vi "MCCDAQ.vi"() -> (0 "error out":errorcluster)   [LabVIEW 2020]
uses:
  Globals/Meas_global.vi
  <vilib>/ULx/Create Channel.llb/ULx Create Channel (AI-Voltage-Basic).vi
  <vilib>/ULx/Timing.llb/ULx Timing (Sample Clock).vi
  <vilib>/ULx/Read.llb/ULx Read (Analog 2D DBL NChan NSamp).vi
  C:/Program Files (x86)/National Instruments/LabVIEW 2020/vi.lib/ULx/ULx_LV.dll
  Sub_vis/Upload Data.ctl
panel:
  out "format string":string
  out "DeviceName":string
  out "FsReq":dbl
  out "FsRead":dbl format="%#_11g"
  out "AuditTrail":string[](array[string])
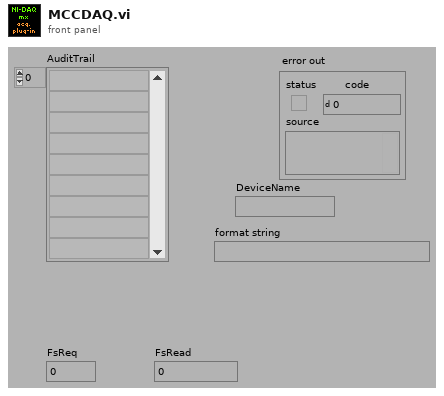
[diagram p1: front panel]
types:
  T1 = typedef "Analysis_info_cluster.ctl" = cluster{"Colour":u32, "Inst type":T2, "Inst name":string, "Symbol":string, "Code name":string, "Extra Info":string, "Inst Array":T3, "Extra Titles":string[], "Extra Values":string[], "U":dbl, "u^2":dbl, "u^3":dbl, "u^4":dbl, "Skew_u":dbl, "Kurt_u":dbl, "Sd Error in Mean":dbl, "% u'/U":dbl, "X":dbl, "Y":dbl, "Z":dbl, "Timescale integral Estimate":dbl, "Sd Error in Variance":dbl, "Calib File":path, "Calib Constants":dbl[], "Output Position":bool, "Stats":enum16{"None", "Basic", "Full"}, "Av Sampling Rate":dbl, "Av No of Samples":dbl, "Total Meas Time (s)":dbl, "ADAM Ch Name":string, "Max value":dbl, "Min value":dbl, "Req Sample Rate Hz":dbl, "Sync Delay Time (s)":dbl, "Ch No":i16, "Device":string, "Use Latest Calib":bool, "Port":string, "Metadata Ch Names":string[], "Metadata Ch Values":string[], "Label":string}
  T2 = typedef "Inst_type.ctl" = enum16{"Raw voltage", "Raw with zero offsetting", "Propeller anemometer", "Pressure Transducer", "Pitot-static tube", "Hot wire", "Cross wire 1", "Cross wire 2", "Generic Linear", "Generic Polynomial", "Generic BackPoly", "Fast FID", "Thermocouple", "Cold wire", "Pulsed Wire", "LDA Vel", "LDA Tran time", "LDA Arr time", "Microphone"}
  T3 = typedef "Instrument_Array.ctl" = enum16{"PWA", "LDA", "Analogue"}
  T4 = typedef "Device ID port info.ctl" = cluster{"Ch No":i16[], "Req Sampling Rate":dbl[], "Port":string, "Index":i32[]}
  T5 = typedef "Upload Data.ctl" = enum16{"Voltage Array", "Time Trace Cluster"}
  T6 = typedef "Rendezvous RefNum" = refnum<k1>
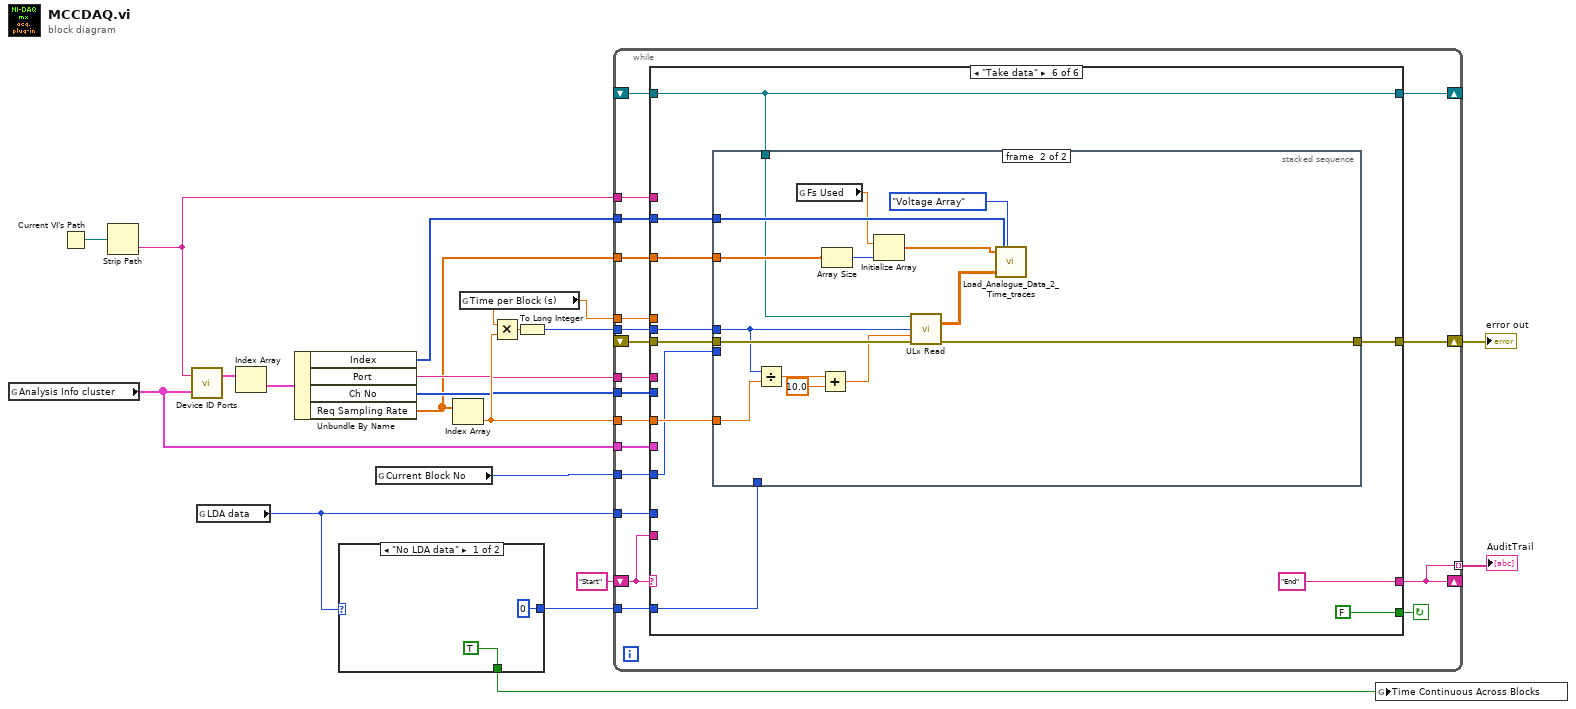
[diagram p0: block diagram]
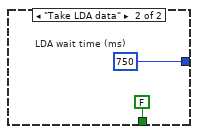
[diagram p2: hidden frame]
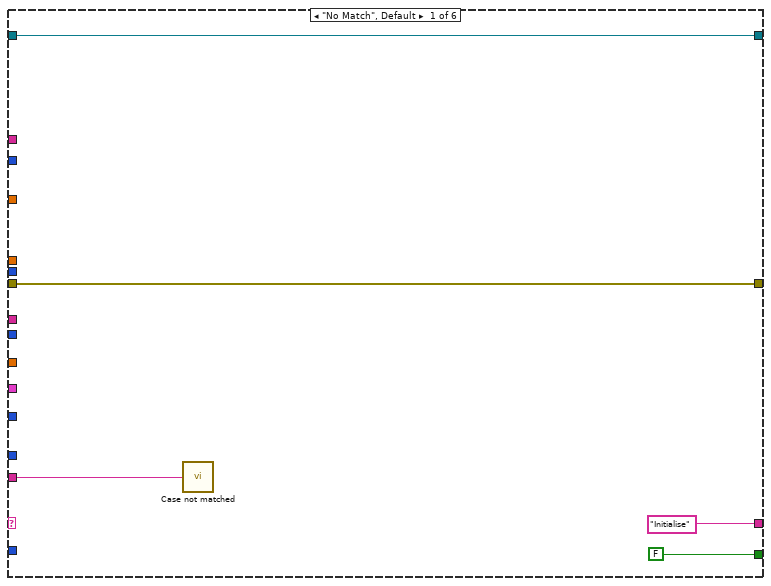
[diagram p3: hidden frame]
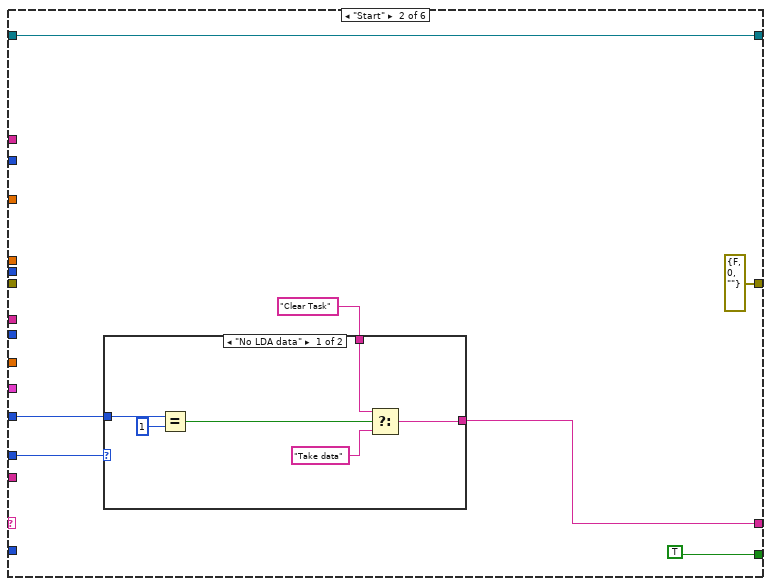
[diagram p4: hidden frame]
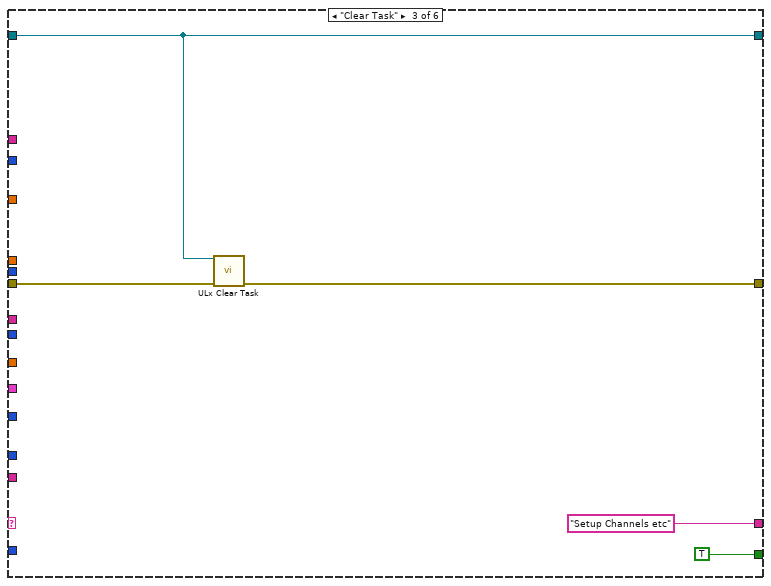
[diagram p6: hidden frame]
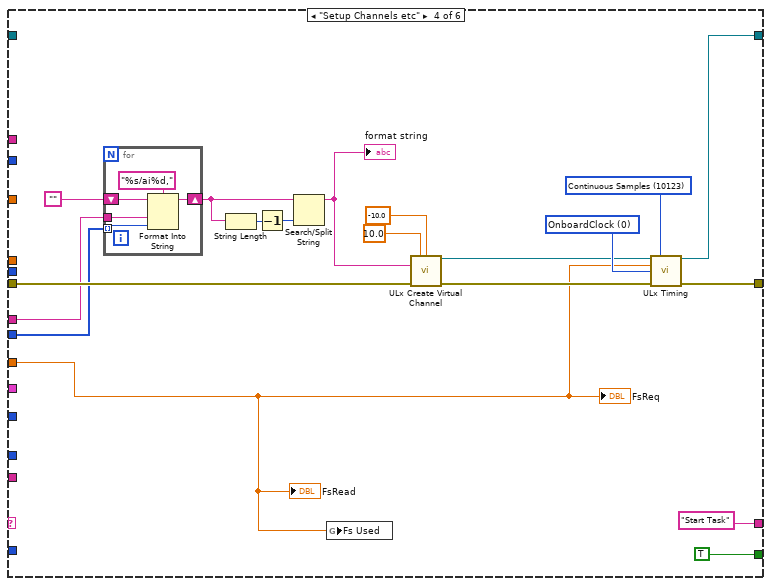
[diagram p7: hidden frame]
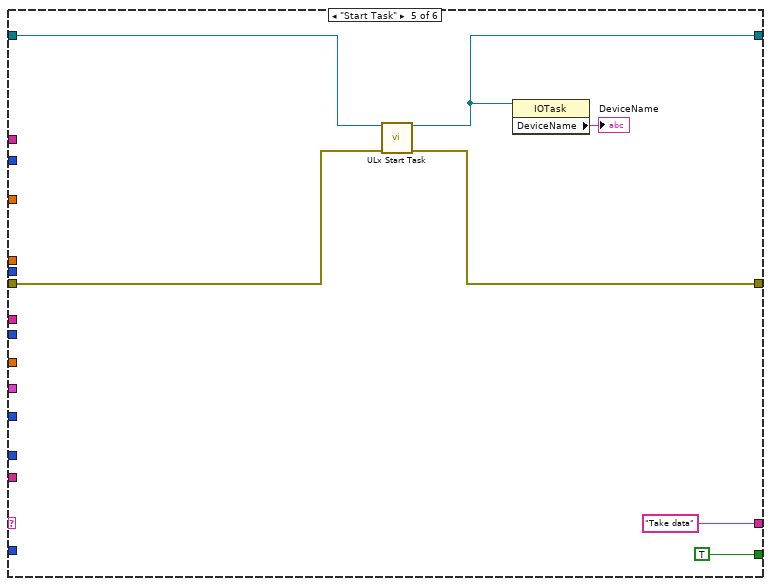
[diagram p8: hidden frame]
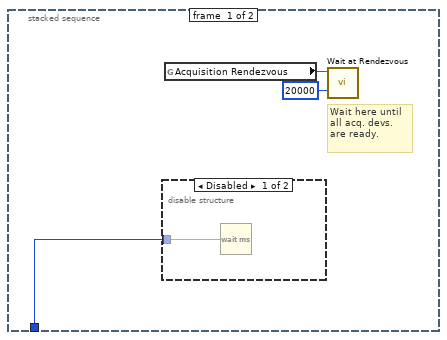
[diagram p9: hidden frame]
diagram:
  n1 = global read "Meas_global.vi" "Analysis Info cluster"() -> (w3:T1[])
  n2 = Current VI's Path() -> (path=w12:path)
  n3 = Strip Path(path=w12) -> (name=w4:string)  [unwired: 1 out]
  n4 = call "Device ID Ports.vi"("Analysis Info cluster"=w3, "Device ID"=w4) -> ("Device port info"=w10:T4[])  [unwired: 1 out]
  n5 = global read "Meas_global.vi" "LDA data"() -> (w19:enum16{"No LDA data", "Take LDA data"})
  n6 = Index Array(array=w10) -> (element=w9:T4)  [unwired: 1 in]
  n7 = Unbundle By Name(w9) -> ("Index"=w7:i32[], "Port"=w8:string, "Ch No"=w6:i16[], "Req Sampling Rate"=w5:dbl[])
  n8 = case shown="\"No LDA data\"" w19 {
    tunnel: [TRUE ("Time Continuous across Blocks") FALSE ("Time Continuous across Blocks")] -> w16
    tunnel: [u32 0 ("LDA wait time (ms)") w23] -> w15
    frame "No LDA data" {
    }
    frame "Take LDA data" {
      w23 = u32 750  # LDA wait time (ms)
    }
  }
  n9 = global read "Meas_global.vi" "Current Block No"() -> (w1:i32)
  n10 = Index Array(array=w5) -> (element=w11:dbl)  [unwired: 1 in]
  n11 = global read "Meas_global.vi" "Time per Block (s)"() -> (w2:dbl)
  n12 = Multiply(x=w2, y=w11) -> (x*y=w13:dbl)
  n13 = To Long Integer(number=w13) -> (32bit integer=w18:i32)
  n14 = while {
    shift-left: "Start" -> [w43]
    shift-right: [w34] -> _
    shift-right: [w38] -> w14
    shift-left: _ -> [w42]
    tunnel: w11 -> [w41]
    tunnel: w18 -> [w40]
    tunnel: w1 -> [w39]
    shift-right: [w37] -> _
    shift-left: _ -> [w36]
    tunnel: w19 -> [w35]
    tunnel: [w34] -> w17 mode=indexing
    tunnel: w15 -> [w33]
    tunnel: w6 -> [w32]
    tunnel: w8 -> [w31]
    tunnel: w5 -> [w30]
    tunnel: w7 -> [w29]
    tunnel: w4 -> [w28]
    tunnel: w3 -> [w27]
    tunnel: w2 -> [w25]
    stop <- w26 continue-if-true
    n15 = case shown="\"Take data\"" w43 {
      tunnel: [FALSE TRUE TRUE TRUE TRUE FALSE] -> w26
      tunnel: ["Initialise" w54 "Setup Channels etc" "Start Task" "Take data" "End"] -> w34
      tunnel: w43 -> [w44 _ _ _ _ _]
      tunnel: [w46 errorcluster {"status"=FALSE, "code"=0, "source"=""} ("error out") w64 w83 w94 w101] -> w38
      tunnel: w42 -> [w46 _ w65 w79 w95 w109]
      tunnel: w41 -> [_ _ _ w78 _ w106]
      tunnel: w40 -> [_ _ _ _ _ w105]
      tunnel: w39 -> [_ w53 _ _ _ w100]
      tunnel: [w45 w50 w63 w77 w92 w99] -> w37
      tunnel: w36 -> [w45 w50 w63 _ w96 w99]
      tunnel: w35 -> [_ w52 _ _ _ _]
      tunnel: w33 -> [_ _ _ _ _ w104]
      tunnel: w32 -> [_ _ _ w76 _ _]
      tunnel: w31 -> [_ _ _ w68 _ _]
      tunnel: w30 -> [_ _ _ _ _ w103]
      tunnel: w29 -> [_ _ _ _ _ w102]
      tunnel: w28 -> [_ _ _ _ _ _]
      tunnel: w27 -> [_ _ _ _ _ _]
      tunnel: w25 -> [_ _ _ _ _ _]
      frame "No Match", Default {
        n16 = call "Case not matched.vi"("Case Name not Matched"=w44) -> ()
      }
      frame "Start" {
        n17 = case shown="\"No LDA data\"" w52 {
          tunnel: "Clear Task" -> [w61 w62]
          tunnel: [w59 w62] -> w54
          tunnel: w53 -> [w58 _]
          frame "No LDA data" {
            n18 = Equal?(x=w58, y=1) -> (x = y?=w56:bool)
            n19 = Select(t=w61, s=w56, f="Take data") -> (s? t:f=w59:string)
          }
          frame "Take LDA data" {
          }
        }
      }
      frame "Clear Task" {
        n20 = call <vilib>:"ULx Clear Task.vi"("task in"=w63, "error in"=w65) -> ("error out"=w64:errorcluster)  [unwired: 13 in]
      }
      frame "Setup Channels etc" {
        w81 = 0 items=["OnboardClock", "ExternalClock", "NoClock"] ("clock source")
        w84 = 10123 items=["Finite Samples"=10178, "Continuous Samples"=10123, "Hardware Timed Single Point"=12522] ("sample mode")
        n21 = for {
          tunnel: w76 -> [w88] mode=indexing
          shift-right: [w89] -> w72
          shift-left: "" -> [w90]
          tunnel: w68 -> [w87]
          n22 = Format Into String(format string="%s/ai%d,", initial string=w90, w87, w88) -> (resulting string=w89:string)  [unwired: 1 in, 1 out]
        }
        n23 = String Length(string=w72) -> (length=w73:i32)
        n24 = Decrement(x=w73) -> (x-1=w71:i32)
        n25 = Search/Split String(string=w72, offset (0)=w71) -> (substring before match=w70:string)  [unwired: 1 in, 2 out]
        "format string" <- w70
        n26 = global write "Meas_global.vi" "Fs Used"(w78) -> ()
        n27 = call-poly <vilib>:"ULx Create Virtual Channel.vi"("maximum value"=10.0, "minimum value"=-10.0, "physical channels"=w70, "error in"=w79) -> ("task out"=w80:refnum<k24>, "error out"=w85:errorcluster)  [unwired: 10 in]
        n28 = call-poly <vilib>:"ULx Timing.vi"("task in"=w80, "sample mode"=w84, "rate"=w78, "clock source"=w81, "error in"=w85) -> ("task out"=w77:refnum<k24>, "error out"=w83:errorcluster)  [unwired: 9 in]
        "FsRead" <- w78
        "FsReq" <- w78
      }
      frame "Start Task" {
        n29 = call <vilib>:"ULx Start Task.vi"("task in"=w96, "error in"=w95) -> ("task out"=w92:refnum<k24>, "error out"=w94:errorcluster)  [unwired: 12 in]
        n30 = property class="IOTask"(reference=w92) -> ("DeviceName"=→"DeviceName":string)  [unwired: 1 in, 2 out]
      }
      frame "Take data" {
        n31 = stacked-sequence {
          tunnel: w109 -> [_ w128]
          tunnel: w106 -> [_ w121]
          tunnel: w105 -> [_ w123]
          tunnel: [_ w127] -> w101
          tunnel: w104 -> [w112 _]
          tunnel: w103 -> [_ w119]
          tunnel: w102 -> [_ w120]
          tunnel: w100 -> [_ _]
          tunnel: w99 -> [_ w115]
          frame #0 {
            # "Wait here until all acq. devs. are ready."
            n32 = disable-structure shown="Disabled" {
              disable-tunnel: w112 -> [w113 _]
              frame Disabled {
                n33 = Wait (ms)(milliseconds to wait=w113) -> ()  [unwired: 1 out]
              }
              frame Enabled {
              }
            }
            n34 = global read "Meas_global.vi" "Acquisition Rendezvous"() -> (w111:T6)
            n35 = call <vilib>:"Wait at Rendezvous.vi"("ms timeout (-1)"=20000, "rendezvous"=w111) -> ()  [unwired: 3 in, 3 out]
          }
          frame #1 {
            n36 = Divide(x=w123, y=w121) -> (x/y=w126:dbl)
            n37 = global read "Meas_global.vi" "Fs Used"() -> (w116:dbl)
            n38 = Add(x=w126, y=10.0) -> (x+y=w124:dbl)
            n39 = Array Size(array=w119) -> (size(s)=w118:i32)
            n40 = Initialize Array(w116, w118) -> (w117:dbl[])
            n41 = call-poly <vilib>:"ULx Read.vi"("task in"=w115, "number of samples per channel"=w123, "timeout"=w124, "error in"=w128) -> ("data"=w122:dbl[][], "error out"=w127:errorcluster)  [unwired: 9 in, 1 out]
            n42 = call "Load_Analogue_Data_2_Time_traces.vi"("Sampling Rate (Hz)"=w117, "Mode"=Upload_Data."Voltage Array", "Index"=w120, "Voltage Array"=w122) -> ()  [unwired: 3 in]
          }
        }
      }
    }
  }
  "error out" <- w14
  "AuditTrail" <- w17
  n43 = global write "Meas_global.vi" "Time Continuous Across Blocks"(w16) -> ()
